vi "rtin_setGpioMode.vi"(8 "error in":errorcluster, 10 "gpio_mode":i32, 11 "connection ID":refnum<k5>) -> (0 "error out":errorcluster, 3 "connection ID":refnum<k5>)   [LabVIEW 2016]
doc: "set the GPIO mode for Mic Mode feature"
panel:
  out "params_cluster":cluster{"gpio_mode":i32}
  in  "Params_cluster":cluster{"integer":i32}
  in  "results_cluster":cluster{"errNo":i32}
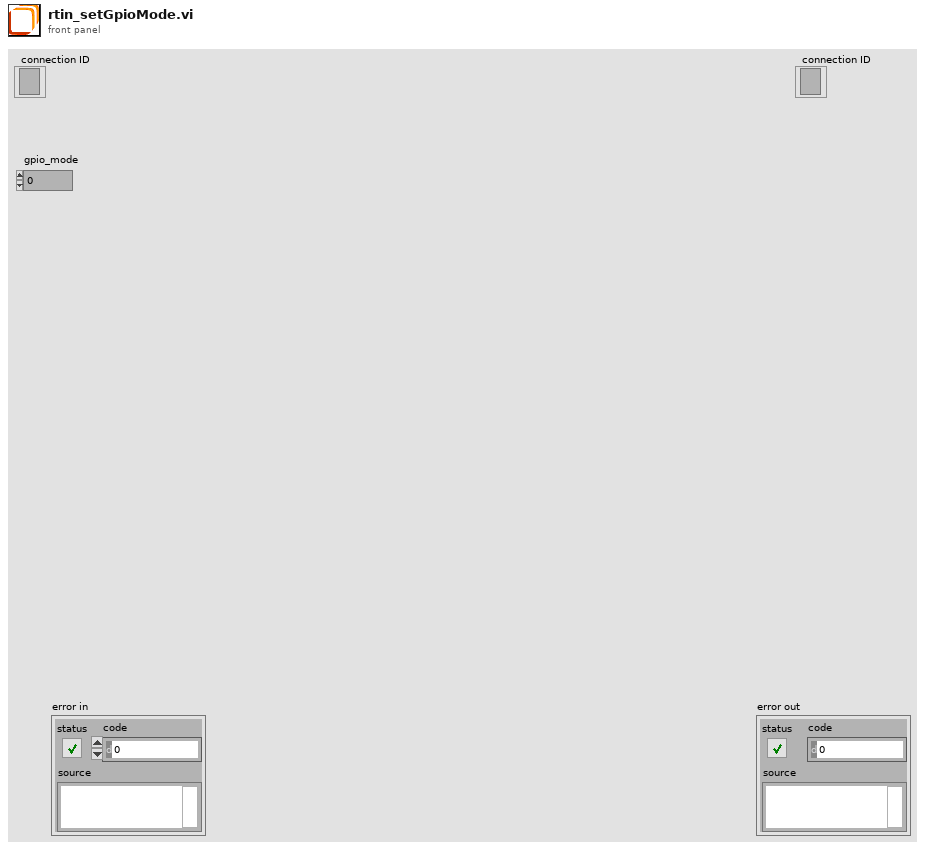
[diagram p1: front panel]
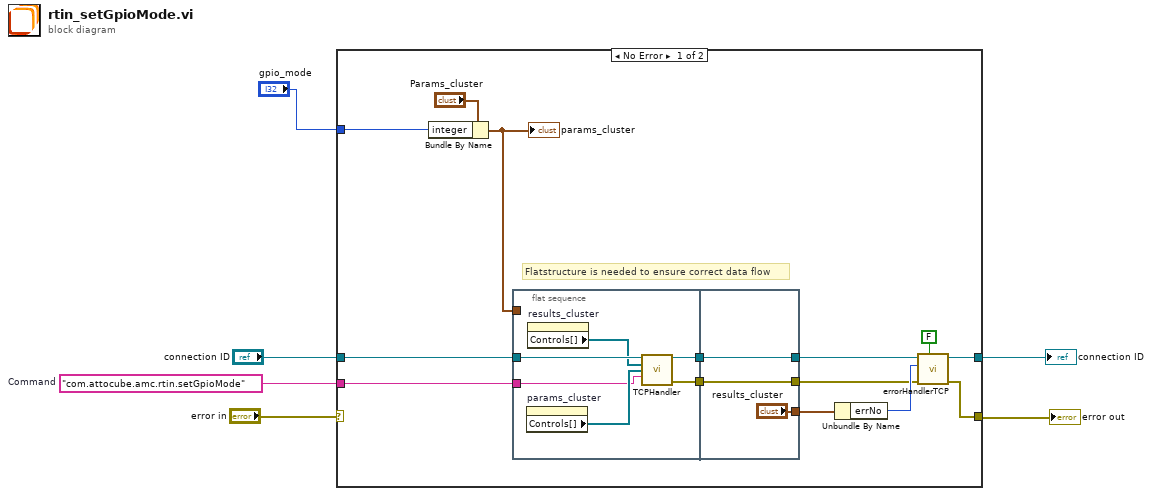
[diagram p0: block diagram]
diagram:
  w2 = "com.attocube.amc.rtin.setGpioMode"  # Command
  n1 = case shown="No Error" "error in" {
    selector: "error in" -> [_ w31]
    tunnel: [w18 w31] -> w6
    tunnel: [w20 w30] -> w5
    tunnel: "connection ID" -> [w17 w30]
    tunnel: w2 -> [w11 _]
    tunnel: "gpio_mode" -> [w7 _]
    frame No Error {
      # "Flatstructure is needed to ensure correct data flow"
      n2 = Bundle By Name(cluster="Params_cluster", "integer"=w7) -> (w8:cluster{"integer":i32})
      "params_cluster" <- w8
      n3 = flat-sequence {
        tunnel: [w25] -> w13
        tunnel: w17 -> [w26]
        tunnel: w11 -> [w22]
        tunnel: [w21] -> w9
        tunnel: w8 -> [_]
        tunnel: ["results_cluster"] -> w14
        tunnel: [w29] -> w16
        tunnel: w13 -> [w29]
        tunnel: [w27] -> w10
        tunnel: w9 -> [w27]
        frame #0 {
          n4 = property on="params_cluster" class="Clust (strict)"() -> ("Controls[]"=w23:refnum<vi>[])  [unwired: 2 in, 2 out]
          n5 = property on="results_cluster" class="Clust (strict)"() -> ("Controls[]"=w24:refnum<vi>[])  [unwired: 2 in, 2 out]
          n6 = call "TCPHandler.vi"("connection ID"=w26, "results_cluster"=w24, "params_cluster"=w23, "method"=w22) -> ("connection ID"=w25:refnum<k5>, "error"=w21:errorcluster)  [unwired: 8 in, 2 out]
        }
        frame #1 {
        }
      }
      n7 = Unbundle By Name(w14) -> ("errNo"=w15:i32)
      n8 = call "errorHandlerTCP.vi"("show popup"=FALSE, "error in"=w10, "error number"=w15, "connection ID"=w16) -> ("error out"=w18:errorcluster, "connection ID"=w20:refnum<k5>)  [unwired: 6 in]
    }
    frame Error {
    }
  }
  "error out" <- w6
  "connection ID" <- w5
